vi "test Parse Unbound Map.vi"() -> (0 "error out":errorcluster, 2 "pass?":bool)   [LabVIEW 2019, in "RESP3 Tests.lvlib"]
uses:
  RESP3 Tests.lvlib
  RESP3/RESP3 Parser/RESP3 Parser.lvclass
  RESP3/types/RESP3 Type.ctl
  2441387c-e5ec-4a74-9e16-53fc1834f06c.vi
  RESP3/types/RESP3 data type attribute.vi
  RESP3/RESP3.lvlib
panel:
  out "RESP3 Value":variant
  out "finished?":bool
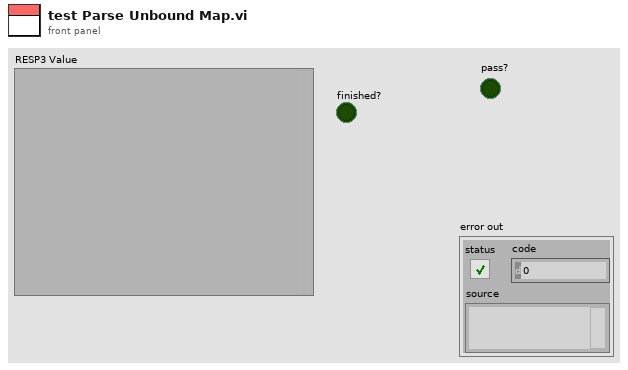
[diagram p1: front panel]
types:
  T1 = typedef "RESP3.lvlib/RESP3 Type.ctl" = enum8{"<0x00>", "<0x01>", "<0x02>", "<0x03>", "<0x04>", "<0x05>", "<0x06>", "<0x07>", "<0x08>", "<0x09>", "<0x0A>", "<0x0B>", "<0x0C>", "<0x0D>", "<0x0E>", "<0x0F>", "<0x10>", "<0x11>", "<0x12>", "<0x13>", "<0x14>", "<0x15>", "<0x16>", "<0x17>", "<0x18>", "<0x19>", "<0x1A>", "<0x1B>", "<0x1C>", "<0x1D>", "<0x1E>", "<0x1F>", "\" \"", "BLOB ERROR", "\"\"\"", "BOOLEAN", "BLOB", "MAP", "\"&\"", "\"'\"", "BIG NUMBER", "\")\"", "ARRAY", "STRING", "DOUBLE", "ERROR", "END", "\"/\"", "\"0\"", "\"1\"", "\"2\"", "\"3\"", "\"4\"", "\"5\"", "\"6\"", "\"7\"", "\"8\"", "\"9\"", "INTEGER", "STREAM", "\"<\"", "VERBATIM STRING", "PUSH", "\"?\"", "\"@\"", "\"A\"", "\"B\"", "\"C\"", "\"D\"", "\"E\"", "\"F\"", "\"G\"", "\"H\"", "\"I\"", "\"J\"", "\"K\"", "\"L\"", "\"M\"", "\"N\"", "\"O\"", "\"P\"", "\"Q\"", "\"R\"", "\"S\"", "\"T\"", "\"U\"", "\"V\"", "\"W\"", "\"X\"", "\"Y\"", "\"Z\"", "\"[\"", "\"\\\"", "\"]\"", "\"^\"", "NULL", "\"`\"", "\"a\"", "\"b\"", "\"c\"", "\"d\"", "\"e\"", "\"f\"", "\"g\"", "\"h\"", "\"i\"", "\"j\"", "\"k\"", "\"l\"", "\"m\"", "\"n\"", "\"o\"", "\"p\"", "\"q\"", "\"r\"", "\"s\"", "\"t\"", "\"u\"", "\"v\"", "\"w\"", "\"x\"", "\"y\"", "\"z\"", "\"{\"", "ATTRIBUTES", "\"}\"", "SET", "<0x7F>", "<0x80>", "<0x81>", "<0x82>", "<0x83>", "<0x84>", "<0x85>", "<0x86>", "<0x87>", "<0x88>", "<0x89>", "<0x8A>", "<0x8B>", "<0x8C>", "<0x8D>", "<0x8E>", "<0x8F>", "<0x90>", "<0x91>", "<0x92>", "<0x93>", "<0x94>", "<0x95>", "<0x96>", "<0x97>", "<0x98>", "<0x99>", "<0x9A>", "<0x9B>", "<0x9C>", "<0x9D>", "<0x9E>", "<0x9F>", "<0xA0>", "<0xA1>", "<0xA2>", "<0xA3>", "<0xA4>", "<0xA5>", "<0xA6>", "<0xA7>", "<0xA8>", "<0xA9>", "<0xAA>", "<0xAB>", "<0xAC>", "<0xAD>", "<0xAE>", "<0xAF>", "<0xB0>", "<0xB1>", "<0xB2>", "<0xB3>", "<0xB4>", "<0xB5>", "<0xB6>", "<0xB7>", "<0xB8>", "<0xB9>", "<0xBA>", "<0xBB>", "<0xBC>", "<0xBD>", "<0xBE>", "<0xBF>", "<0xC0>", "<0xC1>", "<0xC2>", "<0xC3>", "<0xC4>", "<0xC5>", "<0xC6>", "<0xC7>", "<0xC8>", "<0xC9>", "<0xCA>", "<0xCB>", "<0xCC>", "<0xCD>", "<0xCE>", "<0xCF>", "<0xD0>", "<0xD1>", "<0xD2>", "<0xD3>", "<0xD4>", "<0xD5>", "<0xD6>", "<0xD7>", "<0xD8>", "<0xD9>", "<0xDA>", "<0xDB>", "<0xDC>", "<0xDD>", "<0xDE>", "<0xDF>", "<0xE0>", "<0xE1>", "<0xE2>", "<0xE3>", "<0xE4>", "<0xE5>", "<0xE6>", "<0xE7>", "<0xE8>", "<0xE9>", "<0xEA>", "<0xEB>", "<0xEC>", "<0xED>", "<0xEE>", "<0xEF>", "<0xF0>", "<0xF1>", "<0xF2>", "<0xF3>", "<0xF4>", "<0xF5>", "<0xF6>", "<0xF7>", "<0xF8>", "<0xF9>", "<0xFA>", "<0xFB>", "<0xFC>", "<0xFD>", "<0xFE>"}
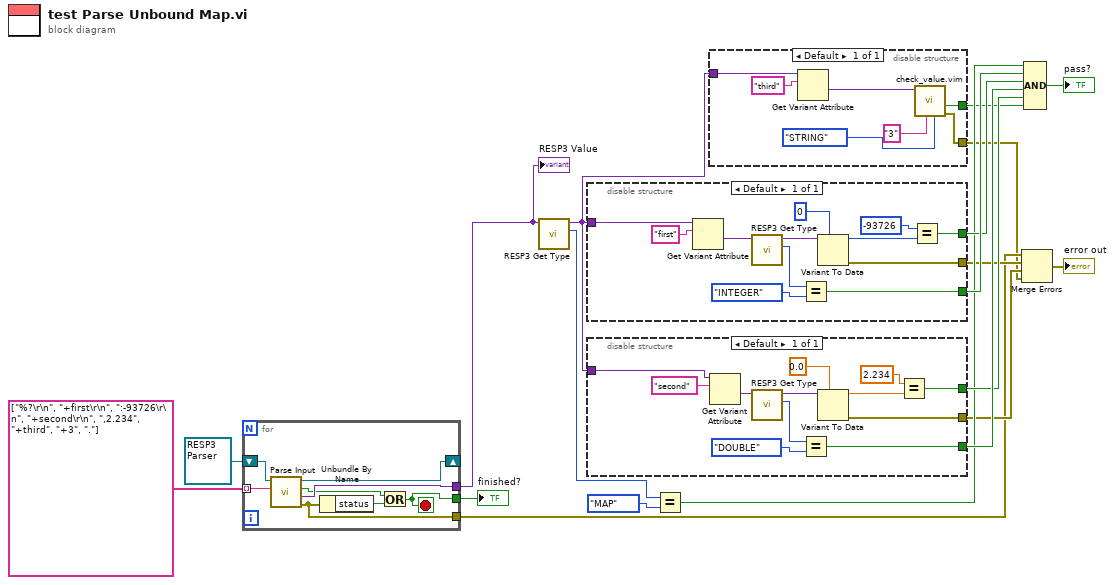
[diagram p0: block diagram]
diagram:
  n1 = for {
    shift-right: [w26] -> _
    shift-left: refnum<class "RESP3 Parser.lvclass"> refnum ("RESP3.lvlib:RESP3 Parser.lvclass") -> [w27]
    tunnel: string[] ["%?\r\n", "+first\r\n", ":-93726\r\n", "+second\r\n", ",2.234", "+third", "+3", "."] -> [w25] mode=indexing
    tunnel: [w24] -> w16
    tunnel: [w22] -> w17
    tunnel: [w20] -> w5
    stop <- w22 stop-if-true
    n2 = call-dynamic "Parse Input.vi"("input line"=w25, "RESP3 Parser in"=w27) -> ("error out"=w20:errorcluster, "RESP3 Value"=w24:variant, "finished?"=w23:bool, "RESP3 Parser out"=w26:refnum<class "RESP3 Parser.lvclass">)  [unwired: 6 in]
    n3 = Unbundle By Name(w20) -> ("status"=w21:bool)
    n4 = Or(x=w23, y=w21) -> (x .or. y?=w22:bool)
  }
  "finished?" <- w17
  "RESP3 Value" <- w16
  n5 = call "RESP3 Get Type.vi"("RESP3 Value in"=w16) -> ("RESP3 Type"=w15:T1, "RESP3 Value out"=w3:variant)  [unwired: 7 in, 2 out]
  n6 = disable-structure shown="Default" {
    disable-tunnel: [w37] -> w12
    disable-tunnel: [w32] -> w11
    disable-tunnel: [w31] -> w7
    disable-tunnel: w3 -> [w29]
    frame Enabled {
      n7 = Get Variant Attribute(Variant=w29, name="first") -> (value=w28:variant)  [unwired: 2 in, 3 out]
      n8 = call "RESP3 Get Type.vi"("RESP3 Value in"=w28) -> ("RESP3 Type"=w38:T1, "RESP3 Value out"=w36:variant)  [unwired: 7 in, 2 out]
      n9 = Equal?(x=w38, y=RESP3_Type."INTEGER") -> (x = y?=w37:bool)
      n10 = Variant To Data(type=i64 0, Variant=w36) -> (data=w34:i64, error out=w31:errorcluster)  [unwired: 1 in]
      n11 = Equal?(x=i64 -93726, y=w34) -> (x = y?=w32:bool)
    }
  }
  n12 = disable-structure shown="Default" {
    disable-tunnel: [w49] -> w10
    disable-tunnel: [w44] -> w9
    disable-tunnel: [w43] -> w6
    disable-tunnel: w3 -> [w42]
    frame Enabled {
      n13 = Get Variant Attribute(Variant=w42, name="second") -> (value=w41:variant)  [unwired: 2 in, 3 out]
      n14 = call "RESP3 Get Type.vi"("RESP3 Value in"=w41) -> ("RESP3 Type"=w50:T1, "RESP3 Value out"=w48:variant)  [unwired: 7 in, 2 out]
      n15 = Equal?(x=w50, y=RESP3_Type."DOUBLE") -> (x = y?=w49:bool)
      n16 = Variant To Data(type=0.0, Variant=w48) -> (data=w46:dbl, error out=w43:errorcluster)  [unwired: 1 in]
      n17 = Equal?(x=2.234, y=w46) -> (x = y?=w44:bool)
    }
  }
  n18 = Equal?(x=w15, y=RESP3_Type."MAP") -> (x = y?=w8:bool)
  n19 = disable-structure shown="Default" {
    disable-tunnel: w3 -> [w58]
    disable-tunnel: [w53] -> w2
    disable-tunnel: [w52] -> w1
    frame Enabled {
      n20 = Get Variant Attribute(Variant=w58, name="third") -> (value=w56:variant)  [unwired: 2 in, 3 out]
      n21 = call "check_value.vim"("expected type"=RESP3_Type."STRING", "expected value"="3", "RESP3 Value"=w56) -> ("error out"=w52:errorcluster, "all OK?"=w53:bool)  [unwired: 5 in, 2 out]
    }
  }
  n22 = Merge Errors(w5, w7, w6, w1) -> (→"error out":errorcluster)
  n23 = Compound Arithmetic op=AND(w8, w12, w11, w10, w9, w2) -> (→"pass?":bool)
